vi "Configure FPGA.vi"(8 "error in":errorcluster, 11 "tCRD in":refnum<class "Aircraft OPCCRD.lvclass">) -> (0 "error out":errorcluster, 3 "tCRD out":refnum<class "Aircraft OPCCRD.lvclass">)   [LabVIEW 2015, in "Aircraft OPCCRD.lvclass"]
uses:
  Aircraft OPCCRD.lvclass
  FPGA/Rate.ctl
  Reusable/Session APIs/File Access/Config Data/Config Data.lvclass
  Reusable/Instrument/Instrument.lvclass/Instrument.ctl
  Reusable/Session APIs/File Access/Config Data/Config Data.lvclass/Config Data.ctl
  Aircraft OPCCRD.lvclass/Aircraft OPCCRD.ctl
  Reusable/CRDS/Main/CRDS.lvclass/CRDS.ctl
  Reusable/Instrument/Read Cfg Session.vi
  Reusable/Session APIs/File Access/Config Data/Accessors/Read Ref.vi
  Accessors/Write FPGA Ref.vi
  Reusable/CRDS/Main/Write NumCoadd.vi
  <vilib>/Utility/config.llb/Read Key (I32).vi
  <vilib>/FPGAPlugInAG/sbRIO-9636/niLvFpga_Open_sbRIO-9636.vi
  <vilib>/Utility/error.llb/Error Cluster From Error Code.vi
  <vilib>/rvi/errors/niLvFpgaAdjustHostInterfaceError.vi
  <vilib>/rvi/interface/common/niFpgaWaitOnOcc.vi
  <userlib>/_Session Fwk/Session - Root.lvclass
  <vilib>/rvi/interface/nirviOpenFPGA/nirviOpenFPGA.xnode
  tFPGA Ref.ctl
  FPGA Bitfiles/Aircraft OPCRD Server.lvbitx
  <vilib>/rvi/interface/nirviReadWriteControl/nirviReadWriteControl.xnode
  <vilib>/rvi/interface/nirviMethod/nirviMethod.xnode
  <vilib>/rvi/errors/niLvFpgaMergeErrorWithErrorCode.vi
  NiFpgaLv.dll
  <vilib>/Utility/config.llb/NI_LVConfig.lvlib
  <vilib>/FPGAPlugInAG/sbRIO-9636/niLvFpga_ConfigureFifo_sbRIO-9636.vi
  <vilib>/FPGAPlugInAG/sbRIO-9636/niLvFpga_StartFifo_sbRIO-9636.vi
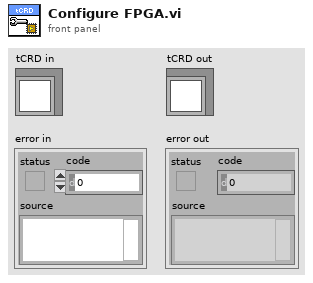
[diagram p1: front panel]
types:
  T1 = typedef "Rate.ctl" = u8
  T2 = typedef "Session - Root.lvclass/Session Handle.ctl" = refnum<data-value>
  T3 = typedef "NI_LVConfig.lvlib/Config Data RefNum.ctl" = refnum<k1>
  T4 = typedef "Aircraft OPCCRD.lvclass/tFPGA Ref.ctl" = refnum<k20>
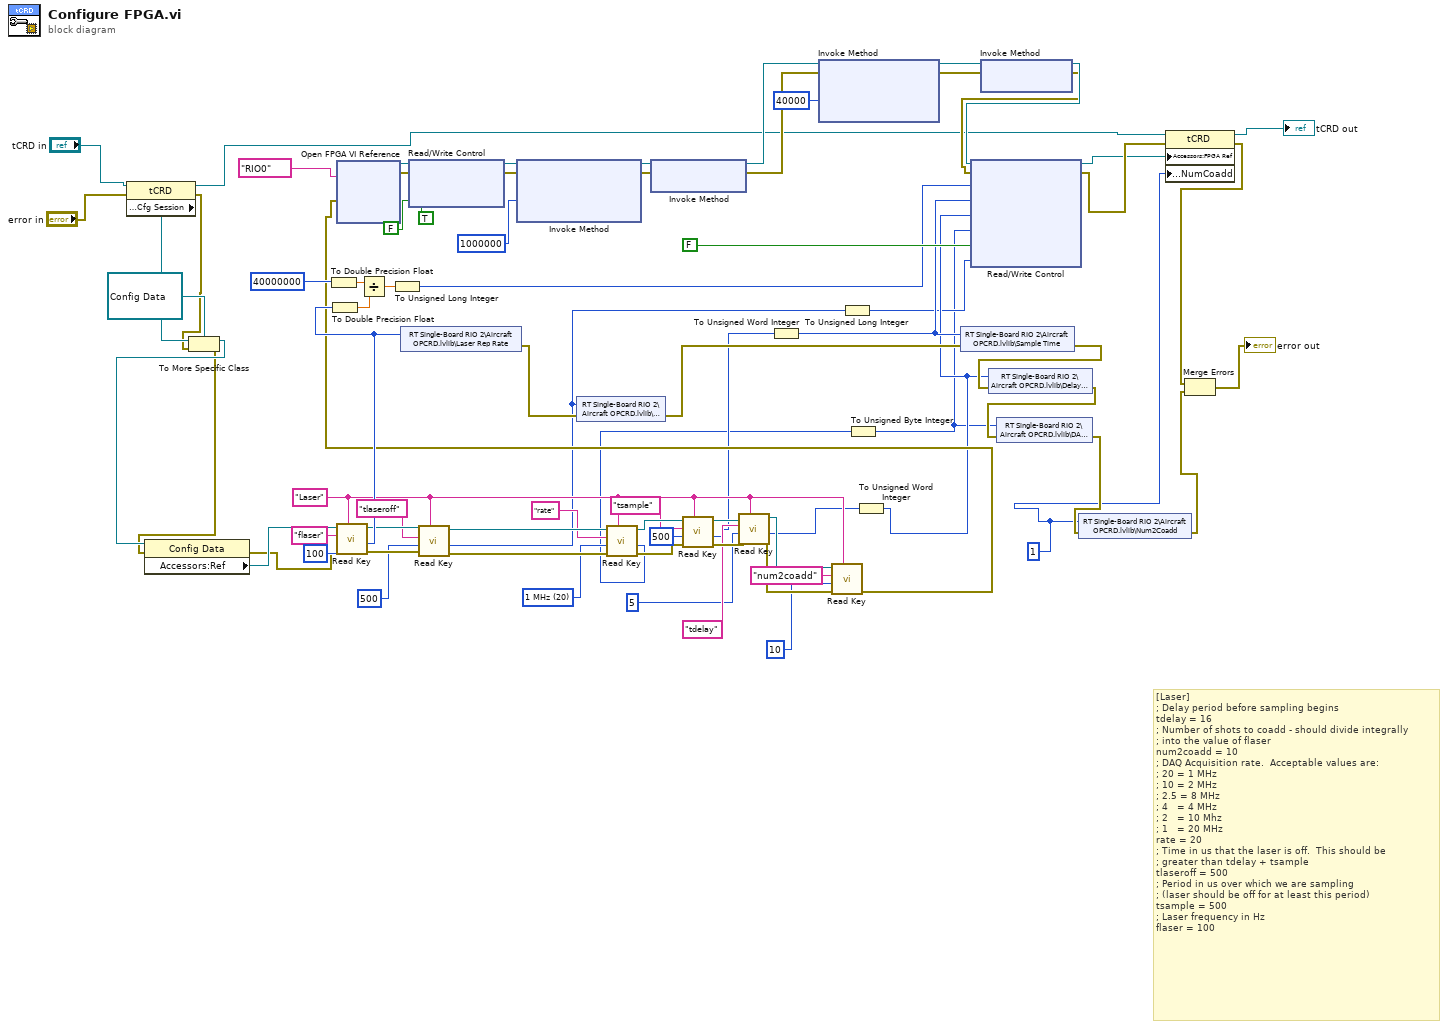
[diagram p0: block diagram]
diagram:
  w17 = 1 ("NumCoadd")
  w30 = "Laser" ("section")
  w42 = T1 20 items=["1 MHz"=20, "2 MHz"=10, "2.5 MHz"=8, "5 MHz"=4, "10 MHz"=2, "20MHz"=1] ("Rate")
  # "[Laser]\n; Delay period before sampling begins\ntdelay = 16\n; Number of shots to coadd - should divide integrally \n; into the value of flaser\nnum2coadd = 10\n; DAQ Acquisition rate.  Acceptable values are:\n; 20 = 1 MHz\n; 10 = 2 MHz\n; 2.5 = 8 MHz\n; 4   = 4 MHz\n; 2   = 10 Mhz\n; 1   = 20 MHz\nrate = 20\n; Time in us that the laser is off.  This should be\n; greater than tdelay + tsample\ntlaseroff = 500\n; Period in us over which we are sampling \n; (laser should be off for at least this period)\ntsample = 500\n; Laser frequency in Hz\nflaser = 100"
  n1 = property class="tCRD"(reference="tCRD in", error in="error in") -> (reference out=w4:refnum<class "Aircraft OPCCRD.lvclass">, error out=w2:errorcluster, "Accessors:Cfg Session"=w8:T2)
  n2 = To More Specific Class(target class=refnum<data-value> refnum, reference=w8, error in=w2) -> (specific class reference=w6:refnum<data-value>, error out=w1:errorcluster)
  n3 = property class="Config Data"(reference=w6, error in=w1) -> (error out=w28:errorcluster, "Accessors:Ref"=w53:T3)  [unwired: 1 out]
  n4 = To Double Precision Float(number=u32 40000000 ("Laser Rep Rate")) -> (double precision float=w70:dbl)
  n5 = call-poly <vilib>:"Read Key.vi"("section"=w30, "error in (no error)"=w28, "default value"=100, "key"="flaser", "refnum"=w53) -> ("error out"=w48:errorcluster, "value"=w51:i32, "refnum out"=w50:T3)  [unwired: 3 in, 1 out]
  n6 = To Double Precision Float(number=w51) -> (double precision float=w68:dbl)
  n7 = Divide(x=w70, y=w68) -> (x/y=w71:dbl)
  n8 = To Unsigned Long Integer(number=w71) -> (unsigned 32bit integer=w67:u32)
  n9 = shared-variable "RT Single-Board RIO 2\\Aircraft OPCRD.lvlib\\Laser Rep Rate"(w51) -> (error out=w61:errorcluster)  [unwired: 1 in]
  n10 = call-poly <vilib>:"Read Key.vi"("section"=w30, "error in (no error)"=w48, "default value"=u32 500 ("LaserOff"), "key"="tlaseroff", "refnum"=w50) -> ("error out"=w44:errorcluster, "value"=w12:i32, "refnum out"=w45:T3)  [unwired: 3 in, 1 out]
  n11 = shared-variable "RT Single-Board RIO 2\\Aircraft OPCRD.lvlib\\LaserOff"(w12, error in=w61) -> (error out=w60:errorcluster)
  n12 = call-poly <vilib>:"Read Key.vi"("section"=w30, "error in (no error)"=w44, "default value"=w42, "key"="rate", "refnum"=w45) -> ("error out"=w40:errorcluster, "value"=w10:i32, "refnum out"=w41:T3)  [unwired: 3 in, 1 out]
  n13 = call-poly <vilib>:"Read Key.vi"("section"=w30, "error in (no error)"=w40, "default value"=500, "key"="tsample", "refnum"=w41) -> ("error out"=w37:errorcluster, "value"=w16:i32, "refnum out"=w38:T3)  [unwired: 3 in, 1 out]
  n14 = call-poly <vilib>:"Read Key.vi"("section"=w30, "error in (no error)"=w37, "default value"=u16 5 ("Delay (us)"), "key"="tdelay", "refnum"=w38) -> ("error out"=w32:errorcluster, "value"=w14:i32, "refnum out"=w33:T3)  [unwired: 3 in, 1 out]
  n15 = To Unsigned Word Integer(number=w16) -> (unsigned 16bit integer=w15:u16)
  n16 = call-poly <vilib>:"Read Key.vi"("section"=w30, "error in (no error)"=w32, "default value"=u8 10 ("Num2Coadd"), "key"="num2coadd", "refnum"=w33) -> ("error out"=w27:errorcluster)  [unwired: 3 in, 3 out]
  n17 = xnode "Open FPGA VI Reference"("error in"=w27, "resource name"=tag "RIO0") -> ("FPGA VI Reference Out"=w76:T4, "error out"=w75:errorcluster)
  n18 = xnode ("Read/Write Control")("FPGA VI Reference In"=w76, "error in"=w75, "Pause Digitizer"=TRUE, "Reverse?"=FALSE) -> ("FPGA VI Reference Out"=w26:T4, "error out"=w25:errorcluster)
  n19 = xnode "Invoke Method"("FPGA VI Reference In"=w26, "error in"=w25, "Requested Depth"=u32 1000000) -> ("FPGA VI Reference Out"=w74:T4, "error out"=w73:errorcluster)  [unwired: 1 out]
  n20 = xnode "Invoke Method"("FPGA VI Reference In"=w74, "error in"=w73) -> ("FPGA VI Reference Out"=w24:T4, "error out"=w23:errorcluster)
  n21 = xnode "Invoke Method"("FPGA VI Reference In"=w24, "error in"=w23, "Requested Depth"=u32 40000) -> ("FPGA VI Reference Out"=w22:T4, "error out"=w21:errorcluster)  [unwired: 1 out]
  n22 = To Unsigned Long Integer(number=w12) -> (unsigned 32bit integer=w11:u32)
  n23 = To Unsigned Byte Integer(number=w10) -> (unsigned 8bit integer=w9:u8)
  n24 = To Unsigned Word Integer(number=w14) -> (unsigned 16bit integer=w13:u16)
  n25 = shared-variable "RT Single-Board RIO 2\\Aircraft OPCRD.lvlib\\Sample Time"(w15, error in=w60) -> (error out=w66:errorcluster)
  n26 = xnode "Invoke Method"("FPGA VI Reference In"=w22, "error in"=w21) -> ("FPGA VI Reference Out"=w20:T4, "error out"=w19:errorcluster)
  n27 = xnode "Read/Write Control"("FPGA VI Reference In"=w20, "error in"=w19, "Cylce (ticks)"=w67, "Sample Time (us)"=w15, "Delay (us)"=w13, "Rate"=w9, "Pause Digitizer"=FALSE, "LaserOff (us)"=w11) -> ("FPGA VI Reference Out"=w54:T4, "error out"=w57:errorcluster)
  n28 = shared-variable "RT Single-Board RIO 2\\Aircraft OPCRD.lvlib\\Delay Time"(w13, error in=w66) -> (error out=w65:errorcluster)
  n29 = shared-variable "RT Single-Board RIO 2\\Aircraft OPCRD.lvlib\\DAQ Rate"(w9, error in=w65) -> (error out=w62:errorcluster)
  n30 = shared-variable "RT Single-Board RIO 2\\Aircraft OPCRD.lvlib\\Num2Coadd"(w17, error in=w62) -> (error out=w59:errorcluster)
  n31 = property class="tCRD"(reference=w4, error in=w57, "Accessors:FPGA Ref"=w54, "Accessors:NumCoadd"=w17) -> (reference out=→"tCRD out":refnum<class "Aircraft OPCCRD.lvclass">, error out=w55:errorcluster)
  n32 = Merge Errors(w55, w59) -> (→"error out":errorcluster)
